vi "close_all_channels.vi"() -> ()   [LabVIEW 2016]
panel:
  out "Channel Name":u16(ring) items=["A1", "A2", "A3", "A4", "A5", "A6", "A7", "A8", "B1", "B2", "B3", "B4", "B5", "B6", "B7", "B8", "C1", "C2", "C3", "C4", "C5", "C6", "C7", "C8"]
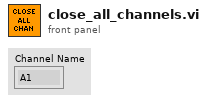
[diagram p1: front panel]
types:
  T1 = enum16{"Release", "Create", "Send", "Wait", "Cancel"}
  T2 = cluster{enum16{"A", "B", "C"}[], enum16{"1", "2", "3", "4", "5", "6", "7", "8"}[], bool[]}
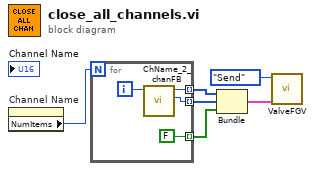
[diagram p0: block diagram]
diagram:
  n1 = property on="Channel Name" class="Ring (strict)"() -> ("NumItems"=w6:u32)  [unwired: 2 in, 2 out]
  n2 = for {
    N: w6 -> [_]
    tunnel: [w9] -> w4 mode=indexing
    tunnel: [w8] -> w5 mode=indexing
    tunnel: [FALSE ("State")] -> w3 mode=indexing
    i -> [w10]
    n3 = call "ChName_2_chanFB.vi"("Channel Name"=w10) -> ("Channel Out"=w9:enum16{"1", "2", "3", "4", "5", "6", "7", "8"}, "Flowboard Out"=w8:enum16{"A", "B", "C"})  [unwired: 9 in]
  }
  n4 = Bundle(w5, w4, w3) -> (w2:T2)  [unwired: 1 in]
  n5 = call "ValveFGV.vi"("Valve Data"=w2, "Action"=T1."Send") -> ()  [unwired: 6 in, 4 out]
